vi "create single curve file path.vi"(0 "base path":path, 1 "Measurement Name":string="-qubitFre", 2 "Sample Name":string, 3 "error in (no error)":errorcluster) -> (5 "file name":string, 7 "data path":path, 8 "para path":path, 10 "error out":errorcluster)   [LabVIEW 2021]
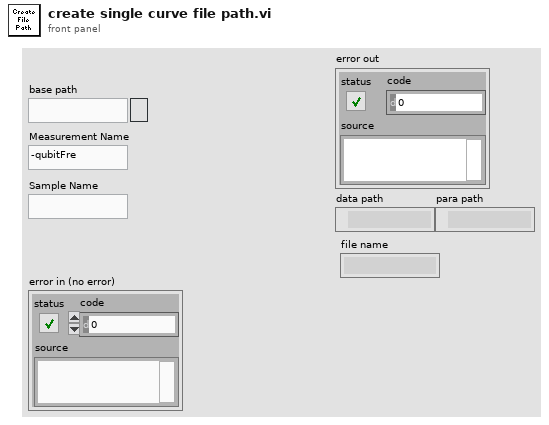
[diagram p1: front panel]
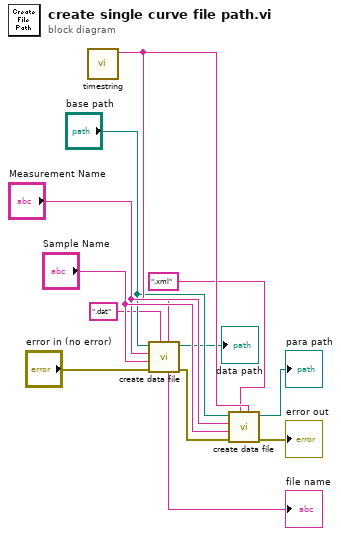
[diagram p0: block diagram]
diagram:
  n1 = call "timestring.vi"() -> ("date/time string"=w10:string)  [unwired: 11 in]
  n2 = call "create data file.vi"("Time"=w10, "Ext name"=".dat", "error in (no error)"="error in (no error)", "Sample Name"="Sample Name", "Measurement Name"="Measurement Name", "base path"="base path") -> ("error out"=w7:errorcluster, "appended path"=→"data path":path, "file name"=→"file name":string)  [unwired: 3 in]
  n3 = call "create data file.vi"("Time"=w10, "Ext name"=".xml", "error in (no error)"=w7, "Sample Name"="Sample Name", "Measurement Name"="Measurement Name", "base path"="base path") -> ("error out"=→"error out":errorcluster, "appended path"=→"para path":path)  [unwired: 3 in, 1 out]
